vi "CMN_ReplaceName.vi"(7 "DBS":string="DBS", 10 "name in":string) -> (2 "name out":string)   [LabVIEW 2016]
uses:
  DBSHAND/private/vis/DatabaseHand_Element_Get(string).vi
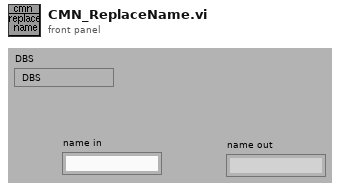
[diagram p1: front panel]
types:
  T1 = typedef "DatabaseHand_RefNum.ctl" = refnum<vi>
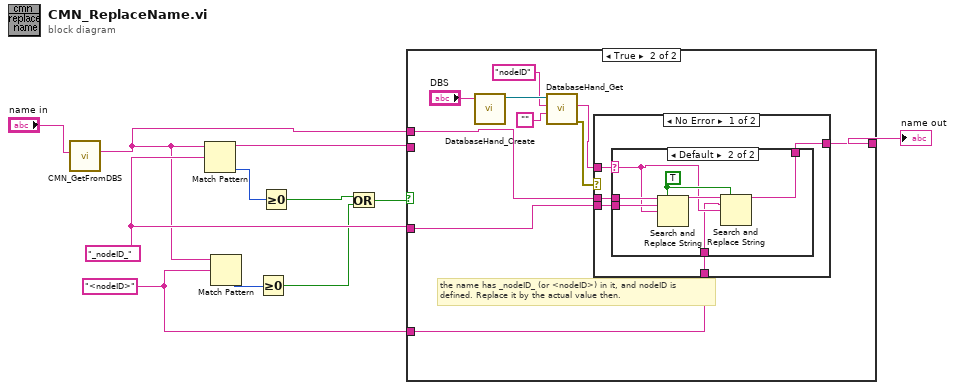
[diagram p0: block diagram]
diagram:
  w1 = "<nodeID>" ("regular expression")
  w8 = "_nodeID_" ("regular expression")
  n1 = call "CMN_GetFromDBS.vi"("str in"="name in") -> ("str out"=w6:string)  [unwired: 10 out]
  n2 = Match Pattern(string=w6, regular expression=w8) -> (before substring=w9:string, offset past match=w11:i32)  [unwired: 3 out]
  n3 = Match Pattern(string=w6, regular expression=w1) -> (offset past match=w5:i32)  [unwired: 4 out]
  n4 = Greater Or Equal To 0?(x=w5) -> (x >= 0?=w2:bool)
  n5 = Greater Or Equal To 0?(x=w11) -> (x >= 0?=w3:bool)
  n6 = Or(x=w3, y=w2) -> (x .or. y?=w4:bool)
  n7 = case shown="True" w4 {
    tunnel: w6 -> [w12 w19]
    tunnel: [w12 w17] -> w10
    tunnel: w9 -> [_ _]
    tunnel: w8 -> [_ w18]
    tunnel: w1 -> [_ w13]
    frame False {
    }
    frame True {
      # "the name has _nodeID_ (or <nodeID>) in it, and nodeID is\ndefined. Replace it by the actual value then."
      n8 = call "DatabaseHand_Create.vi"("Name"="DBS") -> ("Database RefNum out"=w21:T1)  [unwired: 1 in, 9 out]
      n9 = call-poly "DatabaseHand_Get.vi"("default value"="", "name"="nodeID", "Database RefNum in"=w21) -> ("error out"=w14:errorcluster, "value"=w15:string)  [unwired: 2 in, 5 out]
      n10 = case shown="No Error" w14 {
        tunnel: w19 -> [w27 w36]
        tunnel: w18 -> [w26 _]
        tunnel: [w25 w36] -> w17
        tunnel: w15 -> [w24 _]
        tunnel: w13 -> [w23 _]
        frame No Error {
          n11 = case shown="Default" w24 {
            selector: w24 -> [_ w30]
            tunnel: w27 -> [w28 w35]
            tunnel: w26 -> [_ w34]
            tunnel: [w28 w31] -> w25
            tunnel: w23 -> [_ w29]
            frame "", " " {
            }
            frame Default {
              w32 = TRUE ("replace all? (F)")
              n12 = Search and Replace String(replace all?=w32, input string=w35, search string=w34, replace string=w30) -> (result string=w33:string)  [unwired: 1 in, 6 out]
              n13 = Search and Replace String(replace all?=w32, input string=w33, search string=w29, replace string=w30) -> (result string=w31:string)  [unwired: 1 in, 6 out]
            }
          }
        }
        frame Error {
          # "not defined yet.\npass the name intact"
        }
      }
    }
  }
  "name out" <- w10
